vi "URAPI_Jump.vi"(0 "Unique Number":i32, 3 "URAPI Script":T1={"Script"="", "Whiles"=[], "Ifs"=[], "Supress Err"=TRUE, "Errors"=""}) -> (5 "URAPI Script":T1={"Script"="", "Whiles"=[], "Ifs"=[], "Supress Err"=TRUE, "Errors"=""})   [LabVIEW 2012]
doc: "Jumps out of a script, and jumps back in where the \"Land\" partner to this Jump VI is placed. If multiple Jumps/Landings are desired, be sure each pair has matching \"Unique Number\" inputs."
uses:
  <userlib>/BotSpeak/VIs/Direct/URAPI_Control.ctl
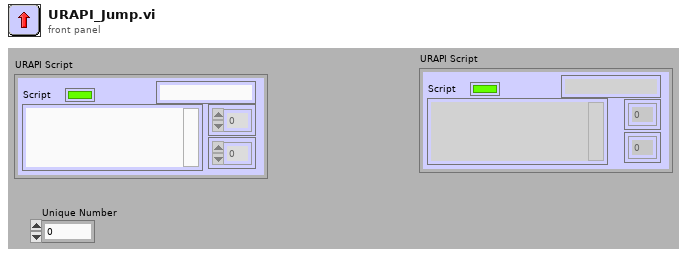
[diagram p1: front panel]
types:
  T1 = typedef "URAPI_Control.ctl" = cluster{"Script":string, "Whiles":u8[], "Ifs":u8[], "Supress Err":bool, "Errors":string}
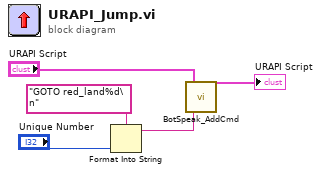
[diagram p0: block diagram]
diagram:
  n1 = Format Into String(format string="GOTO red_land%d\n" ("string"), "Unique Number") -> (resulting string=w3:string)  [unwired: 2 in, 1 out]
  n2 = call <userlib>:"BotSpeak_AddCmd.vi"("String"=w3, "URAPI Script"="URAPI Script") -> ("URAPI Script out"=→"URAPI Script":T1)  [unwired: 1 in]
